vi "4461 - AI AND AI - Read AND Write Uneven.vi"(4 "Reset":bool, 6 "sampling info":cluster{"Fs":dbl, "#s":dbl}={"Fs"=1000.0, "#s"=1000.0} {"Fs" format="%.2p"}, 7 "sample mode":i32(ring)=10178 items=["Finite Samples"=10178, "Continuous Samples"=10123], 8 "error in (no error)":errorcluster, 9 "AO Array":waveform(dbl)[](array[waveform]), 10 "AO Task":refnum<k21>[](array[refnum]), 11 "AI task":refnum<k21>[](array[refnum])=["", ""]) -> (0 "error out":errorcluster, 1 "Input Signals":waveform(dbl)[](array[waveform]))   [LabVIEW 2016]
uses:
  <vilib>/DAQmx/write.llb/DAQmx Write (Analog 1D Wfm NChan NSamp).vi
  <vilib>/DAQmx/read.llb/DAQmx Read (Analog 1D Wfm NChan NSamp).vi
  <vilib>/DAQmx/miscellaneous.llb/DAQmx Fill In Error Info.vi
  <resource>/objmgr/daqmx.rc
panel:
  out "Numeric":i32
  out "AvailSampPerChan 4":u32
  out "AvailSampPerChan 3":u32
  out "AvailSampPerChan 2":u32
  out "AvailSampPerChan 1":u32
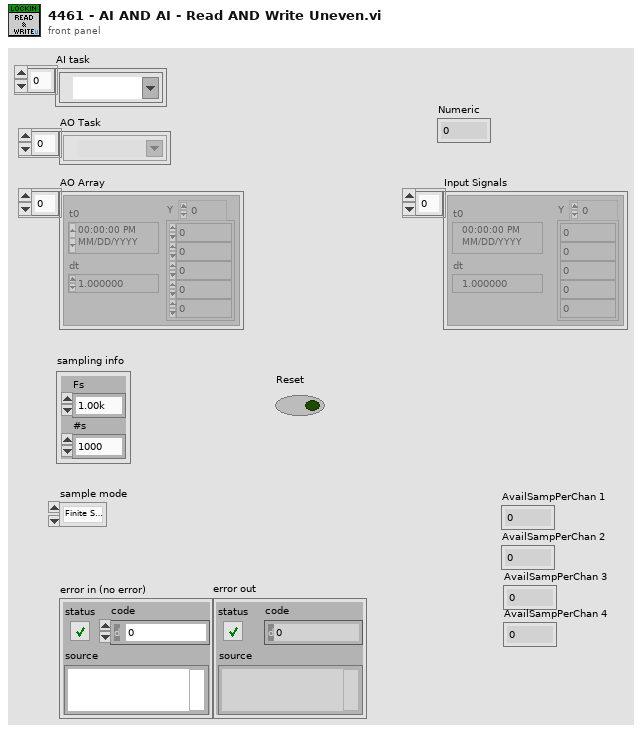
[diagram p1: front panel]
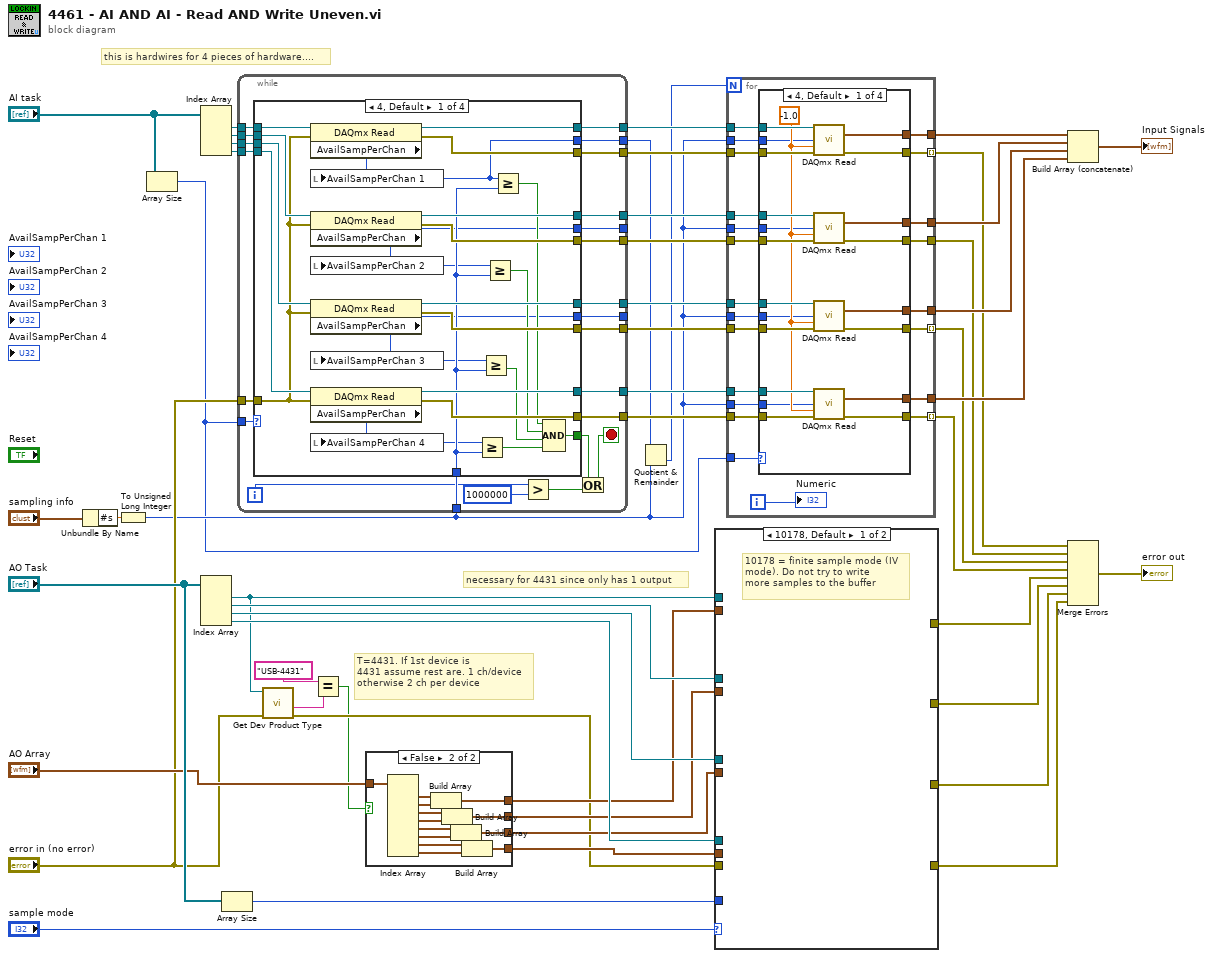
[diagram p0: block diagram]
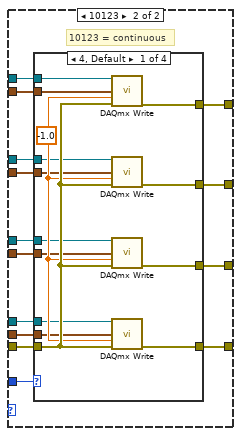
[diagram p2: hidden frame]
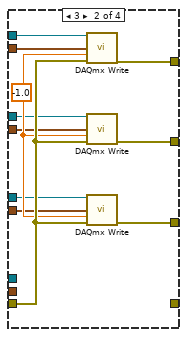
[diagram p3: hidden frame]
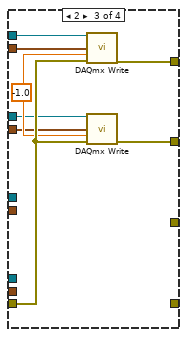
[diagram p4: hidden frame]
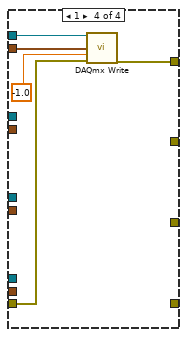
[diagram p5: hidden frame]
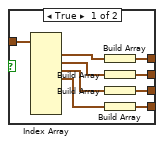
[diagram p6: hidden frame]
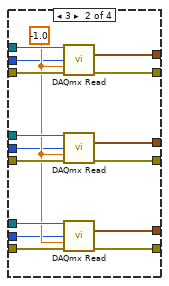
[diagram p7: hidden frame]
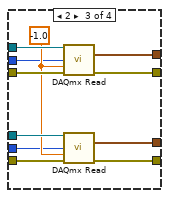
[diagram p8: hidden frame]
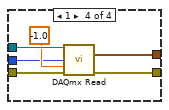
[diagram p9: hidden frame]
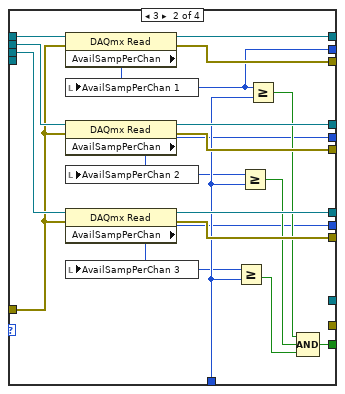
[diagram p10: hidden frame]
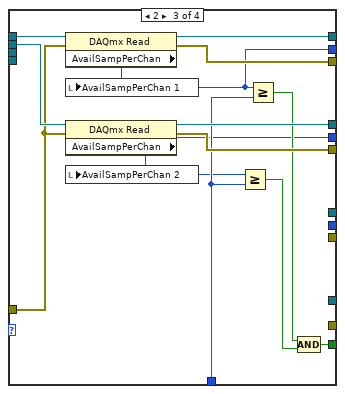
[diagram p11: hidden frame]
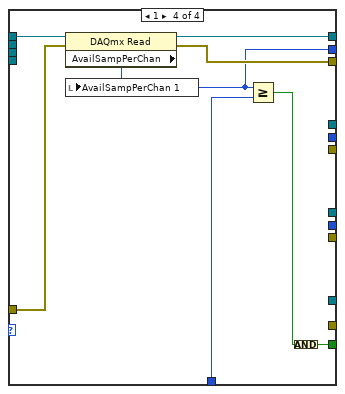
[diagram p12: hidden frame]
diagram:
  # "this is hardwires for 4 pieces of hardware...."
  # "T=4431. If 1st device is \n4431 assume rest are. 1 ch/device\notherwise 2 ch per device"
  # "necessary for 4431 since only has 1 output"
  n1 = Unbundle By Name("sampling info") -> ("#s"=w48:dbl)
  n2 = To Unsigned Long Integer(number=w48) -> (unsigned 32bit integer=w7:u32)
  n3 = Array Size(array="AI task") -> (size(s)=w5:i32)
  n4 = Index Array(array="AI task") -> (element #1=w41:refnum<k21>, element #2=w42:refnum<k21>, element #3=w43:refnum<k21>, element #4=w44:refnum<k21>)  [unwired: 4 in]
  n5 = Index Array(array="AO Task") -> (element #1=w18:refnum<k21>, element #2=w32:refnum<k21>, element #3=w31:refnum<k21>, element #4=w30:refnum<k21>)  [unwired: 4 in]
  n6 = Array Size(array="AO Task") -> (size(s)=w19:i32)
  n7 = while {
    tunnel: w44 -> [w73]
    tunnel: w43 -> [w72]
    tunnel: w42 -> [w71]
    tunnel: w41 -> [w70]
    tunnel: [w69] -> w40
    tunnel: [w68] -> w39
    tunnel: [w67] -> w38
    tunnel: [w66] -> w37
    tunnel: "error in (no error)" -> [w61]
    tunnel: [w65] -> w36
    tunnel: [w64] -> w35
    tunnel: [w63] -> w34
    tunnel: [w62] -> w33
    tunnel: w7 -> [w60]
    tunnel: [w57] -> w20
    tunnel: [w59] -> _
    tunnel: [w58] -> _
    tunnel: w5 -> [w56]
    i -> [w53]
    stop <- w54 stop-if-true
    n8 = case shown="4, Default" w56 {
      tunnel: w73 -> [w96 _ _ _]
      tunnel: w72 -> [w95 w114 _ _]
      tunnel: w71 -> [w94 w113 w127 _]
      tunnel: w70 -> [w93 w112 w126 w135]
      tunnel: [w92 w111 w125 w134] -> w69
      tunnel: [w91 w110 w124 _] -> w68
      tunnel: [w90 w109 _ _] -> w67
      tunnel: [w89 _ _ _] -> w66
      tunnel: [w88 w108 w123 w133] -> w65
      tunnel: [w87 w107 w122 _] -> w64
      tunnel: [w86 w106 _ _] -> w63
      tunnel: [w85 _ _ _] -> w62
      tunnel: w61 -> [w84 w105 w121 w132]
      tunnel: w60 -> [w79 w101 w118 w130]
      tunnel: [w74 w97 w115 w128] -> w55
      tunnel: [w77 w100 _ _] -> w59
      tunnel: [w76 w99 w117 _] -> w58
      tunnel: [w75 w98 w116 w129] -> w57
      frame 4, Default {
        n9 = property class="DAQmx Read"(reference=w93, error in=w84) -> (reference out=w92:refnum<k21>, error out=w88:errorcluster, "AvailSampPerChan"=w75:u32)
        n10 = local write "AvailSampPerChan 1"(w75) -> ()
        n11 = property class="DAQmx Read"(reference=w94, error in=w84) -> (reference out=w91:refnum<k21>, error out=w87:errorcluster, "AvailSampPerChan"=w76:u32)
        n12 = local write "AvailSampPerChan 2"(w76) -> ()
        n13 = property class="DAQmx Read"(reference=w95, error in=w84) -> (reference out=w90:refnum<k21>, error out=w86:errorcluster, "AvailSampPerChan"=w77:u32)
        n14 = local write "AvailSampPerChan 3"(w77) -> ()
        n15 = property class="DAQmx Read"(reference=w96, error in=w84) -> (reference out=w89:refnum<k21>, error out=w85:errorcluster, "AvailSampPerChan"=w78:u32)
        n16 = local write "AvailSampPerChan 4"(w78) -> ()
        n17 = Greater Or Equal?(x=w78, y=w79) -> (x >= y?=w83:bool)
        n18 = Greater Or Equal?(x=w77, y=w79) -> (x >= y?=w82:bool)
        n19 = Greater Or Equal?(x=w76, y=w79) -> (x >= y?=w81:bool)
        n20 = Greater Or Equal?(x=w75, y=w79) -> (x >= y?=w80:bool)
        n21 = Compound Arithmetic op=AND(w80, w81, w82, w83) -> (w74:bool)
      }
      frame 3 {
        n22 = property class="DAQmx Read"(reference=w112, error in=w105) -> (reference out=w111:refnum<k21>, error out=w108:errorcluster, "AvailSampPerChan"=w98:u32)
        n23 = local write "AvailSampPerChan 1"(w98) -> ()
        n24 = property class="DAQmx Read"(reference=w113, error in=w105) -> (reference out=w110:refnum<k21>, error out=w107:errorcluster, "AvailSampPerChan"=w99:u32)
        n25 = local write "AvailSampPerChan 2"(w99) -> ()
        n26 = property class="DAQmx Read"(reference=w114, error in=w105) -> (reference out=w109:refnum<k21>, error out=w106:errorcluster, "AvailSampPerChan"=w100:u32)
        n27 = local write "AvailSampPerChan 3"(w100) -> ()
        n28 = Greater Or Equal?(x=w100, y=w101) -> (x >= y?=w104:bool)
        n29 = Greater Or Equal?(x=w99, y=w101) -> (x >= y?=w103:bool)
        n30 = Greater Or Equal?(x=w98, y=w101) -> (x >= y?=w102:bool)
        n31 = Compound Arithmetic op=AND(w102, w103, w104) -> (w97:bool)
      }
      frame 2 {
        n32 = property class="DAQmx Read"(reference=w126, error in=w121) -> (reference out=w125:refnum<k21>, error out=w123:errorcluster, "AvailSampPerChan"=w116:u32)
        n33 = local write "AvailSampPerChan 1"(w116) -> ()
        n34 = property class="DAQmx Read"(reference=w127, error in=w121) -> (reference out=w124:refnum<k21>, error out=w122:errorcluster, "AvailSampPerChan"=w117:u32)
        n35 = local write "AvailSampPerChan 2"(w117) -> ()
        n36 = Greater Or Equal?(x=w117, y=w118) -> (x >= y?=w120:bool)
        n37 = Greater Or Equal?(x=w116, y=w118) -> (x >= y?=w119:bool)
        n38 = Compound Arithmetic op=AND(w119, w120) -> (w115:bool)
      }
      frame 1 {
        n39 = property class="DAQmx Read"(reference=w135, error in=w132) -> (reference out=w134:refnum<k21>, error out=w133:errorcluster, "AvailSampPerChan"=w129:u32)
        n40 = local write "AvailSampPerChan 1"(w129) -> ()
        n41 = Greater Or Equal?(x=w129, y=w130) -> (x >= y?=w131:bool)
        n42 = Compound Arithmetic op=AND(w131) -> (w128:bool)
      }
    }
    n43 = Greater?(x=w53, y=1000000) -> (0:w51:bool)
    n44 = Or(x=w55, y=w51) -> (x .or. y?=w54:bool)
  }
  n45 = call "Get Dev Product Type.vi"("error in (no error)"="error in (no error)", "Refnum in"=w18) -> ("error out"=w9:errorcluster, "ProductType"=w11:string)  [unwired: 6 in, 2 out]
  n46 = Equal?(x="USB-4431" ("ProductType"), y=w11) -> (x = y?=w6:bool)
  n47 = case shown="False" w6 {
    tunnel: [w144 w150] -> w14
    tunnel: [w143 w149] -> w15
    tunnel: [w142 w148] -> w16
    tunnel: [w140 w146] -> w13
    tunnel: "AO Array" -> [w139 w145]
    frame True {
      n48 = Index Array(array=w139) -> (element #1=w141:waveform(dbl), element #2=w138:waveform(dbl), element #3=w137:waveform(dbl), element #4=w136:waveform(dbl))  [unwired: 8 in, 4 out]
      n49 = Build Array(w141) -> (w140:waveform(dbl)[])
      n50 = Build Array(w138) -> (w144:waveform(dbl)[])
      n51 = Build Array(w137) -> (w143:waveform(dbl)[])
      n52 = Build Array(w136) -> (w142:waveform(dbl)[])
    }
    frame False {
      n53 = Index Array(array=w145) -> (element #1=w147:waveform(dbl), element #2=w157:waveform(dbl), element #3=w156:waveform(dbl), element #4=w155:waveform(dbl), element #5=w154:waveform(dbl), element #6=w153:waveform(dbl), element #7=w152:waveform(dbl), element #8=w151:waveform(dbl))  [unwired: 8 in]
      n54 = Build Array(w147, w157) -> (w146:waveform(dbl)[])
      n55 = Build Array(w156, w155) -> (w150:waveform(dbl)[])
      n56 = Build Array(w154, w153) -> (w149:waveform(dbl)[])
      n57 = Build Array(w152, w151) -> (w148:waveform(dbl)[])
    }
  }
  n58 = Quotient & Remainder(x=w20, y=w7) -> (floor(x/y)=w21:u32)  [unwired: 1 out]
  n59 = case shown="10178, Default" "sample mode" {
    tunnel: w32 -> [_ w171]
    tunnel: w31 -> [_ w170]
    tunnel: w30 -> [_ w169]
    tunnel: [_ w168] -> w29
    tunnel: [_ w167] -> w28
    tunnel: [_ w166] -> w27
    tunnel: [_ w165] -> w26
    tunnel: w19 -> [_ w164]
    tunnel: w18 -> [_ w163]
    tunnel: w16 -> [_ w162]
    tunnel: w15 -> [_ w161]
    tunnel: w14 -> [_ w160]
    tunnel: w13 -> [_ w159]
    tunnel: w9 -> [_ w158]
    frame 10178, Default {
      # "10178 = finite sample mode (IV\nmode). Do not try to write\nmore samples to the buffer"
    }
    frame 10123 {
      # "10123 = continuous"
      n60 = case shown="4, Default" w164 {
        tunnel: w158 -> [w185 w196 w204 w209]
        tunnel: w171 -> [w183 w194 w202 _]
        tunnel: w170 -> [w182 w193 _ _]
        tunnel: w169 -> [w181 _ _ _]
        tunnel: w160 -> [w180 w192 w201 _]
        tunnel: w161 -> [w179 w191 _ _]
        tunnel: w162 -> [w178 _ _ _]
        tunnel: [w177 w190 w200 w207] -> w168
        tunnel: [w176 w189 w199 _] -> w167
        tunnel: [w175 w188 _ _] -> w166
        tunnel: [w174 _ _ _] -> w165
        tunnel: w163 -> [w173 w187 w198 w206]
        tunnel: w159 -> [w172 w186 w197 w205]
        frame 4, Default {
          w184 = -1.0 ("timeout")
          n61 = call-poly <vilib>:"DAQmx Write.vi"("task/channels in"=w173, "data"=w172, "timeout"=w184, "error in"=w185) -> ("error out"=w177:errorcluster)  [unwired: 9 in, 2 out]
          n62 = call-poly <vilib>:"DAQmx Write.vi"("task/channels in"=w183, "data"=w180, "timeout"=w184, "error in"=w185) -> ("error out"=w176:errorcluster)  [unwired: 9 in, 2 out]
          n63 = call-poly <vilib>:"DAQmx Write.vi"("task/channels in"=w182, "data"=w179, "timeout"=w184, "error in"=w185) -> ("error out"=w175:errorcluster)  [unwired: 9 in, 2 out]
          n64 = call-poly <vilib>:"DAQmx Write.vi"("task/channels in"=w181, "data"=w178, "timeout"=w184, "error in"=w185) -> ("error out"=w174:errorcluster)  [unwired: 9 in, 2 out]
        }
        frame 3 {
          w195 = -1.0 ("timeout")
          n65 = call-poly <vilib>:"DAQmx Write.vi"("task/channels in"=w187, "data"=w186, "timeout"=w195, "error in"=w196) -> ("error out"=w190:errorcluster)  [unwired: 9 in, 2 out]
          n66 = call-poly <vilib>:"DAQmx Write.vi"("task/channels in"=w194, "data"=w192, "timeout"=w195, "error in"=w196) -> ("error out"=w189:errorcluster)  [unwired: 9 in, 2 out]
          n67 = call-poly <vilib>:"DAQmx Write.vi"("task/channels in"=w193, "data"=w191, "timeout"=w195, "error in"=w196) -> ("error out"=w188:errorcluster)  [unwired: 9 in, 2 out]
        }
        frame 2 {
          w203 = -1.0 ("timeout")
          n68 = call-poly <vilib>:"DAQmx Write.vi"("task/channels in"=w198, "data"=w197, "timeout"=w203, "error in"=w204) -> ("error out"=w200:errorcluster)  [unwired: 9 in, 2 out]
          n69 = call-poly <vilib>:"DAQmx Write.vi"("task/channels in"=w202, "data"=w201, "timeout"=w203, "error in"=w204) -> ("error out"=w199:errorcluster)  [unwired: 9 in, 2 out]
        }
        frame 1 {
          n70 = call-poly <vilib>:"DAQmx Write.vi"("task/channels in"=w206, "data"=w205, "timeout"=-1.0, "error in"=w209) -> ("error out"=w207:errorcluster)  [unwired: 9 in, 2 out]
        }
      }
    }
  }
  n71 = for {
    N: w21 -> [_]
    tunnel: w40 -> [w231]
    tunnel: w39 -> [w230]
    tunnel: w38 -> [w229]
    tunnel: w37 -> [w228]
    tunnel: w36 -> [w227]
    tunnel: w35 -> [w226]
    tunnel: w34 -> [w225]
    tunnel: w33 -> [w224]
    tunnel: [w223] -> w25
    tunnel: [w222] -> w24
    tunnel: [w221] -> w23
    tunnel: [w220] -> w22
    tunnel: w7 -> [w219]
    tunnel: w7 -> [w218]
    tunnel: w7 -> [w217]
    tunnel: w7 -> [w216]
    tunnel: [w215] -> w2 mode=indexing
    tunnel: [w214] -> w3
    tunnel: [w213] -> w4 mode=indexing
    tunnel: [w212] -> w1 mode=indexing
    tunnel: w5 -> [w210]
    i -> [w211]
    n72 = case shown="4, Default" w210 {
      tunnel: w231 -> [w252 w268 w279 w285]
      tunnel: w230 -> [w251 w267 w278 _]
      tunnel: w229 -> [w250 w266 _ _]
      tunnel: w228 -> [w249 _ _ _]
      tunnel: w227 -> [w248 w265 w277 w284]
      tunnel: w226 -> [w247 w264 w276 _]
      tunnel: w225 -> [w246 w263 _ _]
      tunnel: w224 -> [w245 _ _ _]
      tunnel: [w243 w261 w274 _] -> w223
      tunnel: [w242 w260 w273 w282] -> w222
      tunnel: [w241 w259 _ _] -> w221
      tunnel: [w240 _ _ _] -> w220
      tunnel: w219 -> [w239 _ _ _]
      tunnel: w218 -> [w238 w258 w272 w281]
      tunnel: w217 -> [w237 w257 _ _]
      tunnel: w216 -> [w236 w256 w271 _]
      tunnel: [w235 w255 w270 w280] -> w215
      tunnel: [w234 w254 w269 _] -> w214
      tunnel: [w233 w253 _ _] -> w213
      tunnel: [w232 _ _ _] -> w212
      frame 4, Default {
        w244 = -1.0 ("timeout")
        n73 = call-poly <vilib>:"DAQmx Read.vi"("task/channels in"=w252, "number of samples per channel"=w238, "timeout"=w244, "error in"=w248) -> ("data"=w242:waveform(dbl)[], "error out"=w235:errorcluster)  [unwired: 9 in, 1 out]
        n74 = call-poly <vilib>:"DAQmx Read.vi"("task/channels in"=w251, "number of samples per channel"=w236, "timeout"=w244, "error in"=w247) -> ("data"=w243:waveform(dbl)[], "error out"=w234:errorcluster)  [unwired: 9 in, 1 out]
        n75 = call-poly <vilib>:"DAQmx Read.vi"("task/channels in"=w250, "number of samples per channel"=w237, "timeout"=w244, "error in"=w246) -> ("data"=w241:waveform(dbl)[], "error out"=w233:errorcluster)  [unwired: 9 in, 1 out]
        n76 = call-poly <vilib>:"DAQmx Read.vi"("task/channels in"=w249, "number of samples per channel"=w239, "timeout"=w244, "error in"=w245) -> ("data"=w240:waveform(dbl)[], "error out"=w232:errorcluster)  [unwired: 9 in, 1 out]
      }
      frame 3 {
        w262 = -1.0 ("timeout")
        n77 = call-poly <vilib>:"DAQmx Read.vi"("task/channels in"=w268, "number of samples per channel"=w258, "timeout"=w262, "error in"=w265) -> ("data"=w260:waveform(dbl)[], "error out"=w255:errorcluster)  [unwired: 9 in, 1 out]
        n78 = call-poly <vilib>:"DAQmx Read.vi"("task/channels in"=w267, "number of samples per channel"=w256, "timeout"=w262, "error in"=w264) -> ("data"=w261:waveform(dbl)[], "error out"=w254:errorcluster)  [unwired: 9 in, 1 out]
        n79 = call-poly <vilib>:"DAQmx Read.vi"("task/channels in"=w266, "number of samples per channel"=w257, "timeout"=w262, "error in"=w263) -> ("data"=w259:waveform(dbl)[], "error out"=w253:errorcluster)  [unwired: 9 in, 1 out]
      }
      frame 2 {
        w275 = -1.0 ("timeout")
        n80 = call-poly <vilib>:"DAQmx Read.vi"("task/channels in"=w279, "number of samples per channel"=w272, "timeout"=w275, "error in"=w277) -> ("data"=w273:waveform(dbl)[], "error out"=w270:errorcluster)  [unwired: 9 in, 1 out]
        n81 = call-poly <vilib>:"DAQmx Read.vi"("task/channels in"=w278, "number of samples per channel"=w271, "timeout"=w275, "error in"=w276) -> ("data"=w274:waveform(dbl)[], "error out"=w269:errorcluster)  [unwired: 9 in, 1 out]
      }
      frame 1 {
        n82 = call-poly <vilib>:"DAQmx Read.vi"("task/channels in"=w285, "number of samples per channel"=w281, "timeout"=-1.0, "error in"=w284) -> ("data"=w282:waveform(dbl)[], "error out"=w280:errorcluster)  [unwired: 9 in, 1 out]
      }
    }
    "Numeric" <- w211
  }
  n83 = Build Array (concatenate)(w24, w25, w23, w22) -> (→"Input Signals":waveform(dbl)[])
  n84 = Merge Errors(w2, w3, w4, w1, w29, w28, w27, w26) -> (→"error out":errorcluster)
